vi "String to Access Level.vi"(1 "String":string) -> (0 "Access":T1)   [LabVIEW 2016, in "UserPwd DB.lvlib" / "UserPwd DB.lvclass"]
uses:
  <userlib>/Common Components/UserPwd DB/UserPwd DB/UserPwd DB.lvclass
  <userlib>/Common Components/UserPwd DB/UserPwd DB/Access Level.ctl
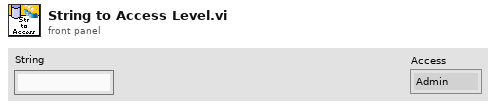
[diagram p1: front panel]
types:
  T1 = typedef "UserPwd DB.lvlib/UserPwd DB.lvclass/Access Level.ctl" = enum16{"Admin", "User lv1", "User lv2", "User lv3", "User lv4", "User lv5", "User lv6", "User lv7", "User lv8", "User lv9", "Guest"}
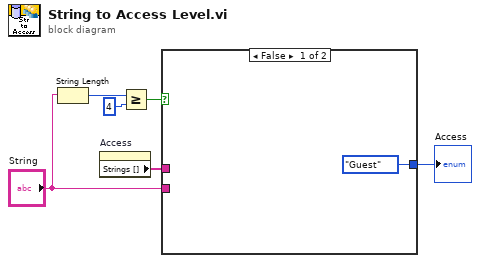
[diagram p0: block diagram]
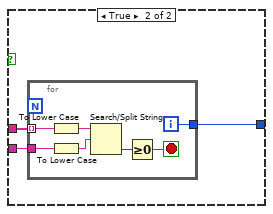
[diagram p2: hidden frame]
diagram:
  n1 = String Length(string="String") -> (length=w3:i32)
  n2 = property on="Access" class="Enum (strict)"() -> ("Strings []"=w6:string[])  [unwired: 2 in, 2 out]
  n3 = Greater Or Equal?(x=w3, y=4) -> (x >= y?=w1:bool)
  n4 = case shown="False" w1 {
    tunnel: w6 -> [_ w10]
    tunnel: [Access_Level."Guest" ("Access") w9] -> w5
    tunnel: "String" -> [_ w8]
    frame False {
    }
    frame True {
      n5 = for {
        tunnel: w10 -> [w17] mode=indexing
        tunnel: w8 -> [w16]
        tunnel: [w11] -> w9
        i -> [w11]
        stop <- w12 stop-if-true
        n6 = To Lower Case(string=w17) -> (all lower case string=w15:string)
        n7 = To Lower Case(string=w16) -> (all lower case string=w14:string)
        n8 = Search/Split String(string=w15, search string/char (-)=w14) -> (offset of match=w13:i32)  [unwired: 1 in, 2 out]
        n9 = Greater Or Equal To 0?(x=w13) -> (x >= 0?=w12:bool)
      }
    }
  }
  "Access" <- w5
